vi "02.4 Transfering Data Through Queues.vi"() -> ()   [LabVIEW 2019]
uses:
  <extravilib>/ChannelInstances/Tag-bool.lvlib
panel:
  in  "Stop":bool
  in  "Process Speed Rate (%)":u32(slide) scale=10.0..200.0
  out "# of elements in Queue":i32
  out "Dequeued data":dbl
  in  "Enqueue Data":bool
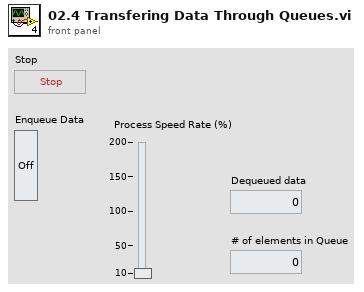
[diagram p1: front panel]
types:
  T1 = typedef "Tag-bool.lvlib/))Channel.ctl" = refnum<queue>
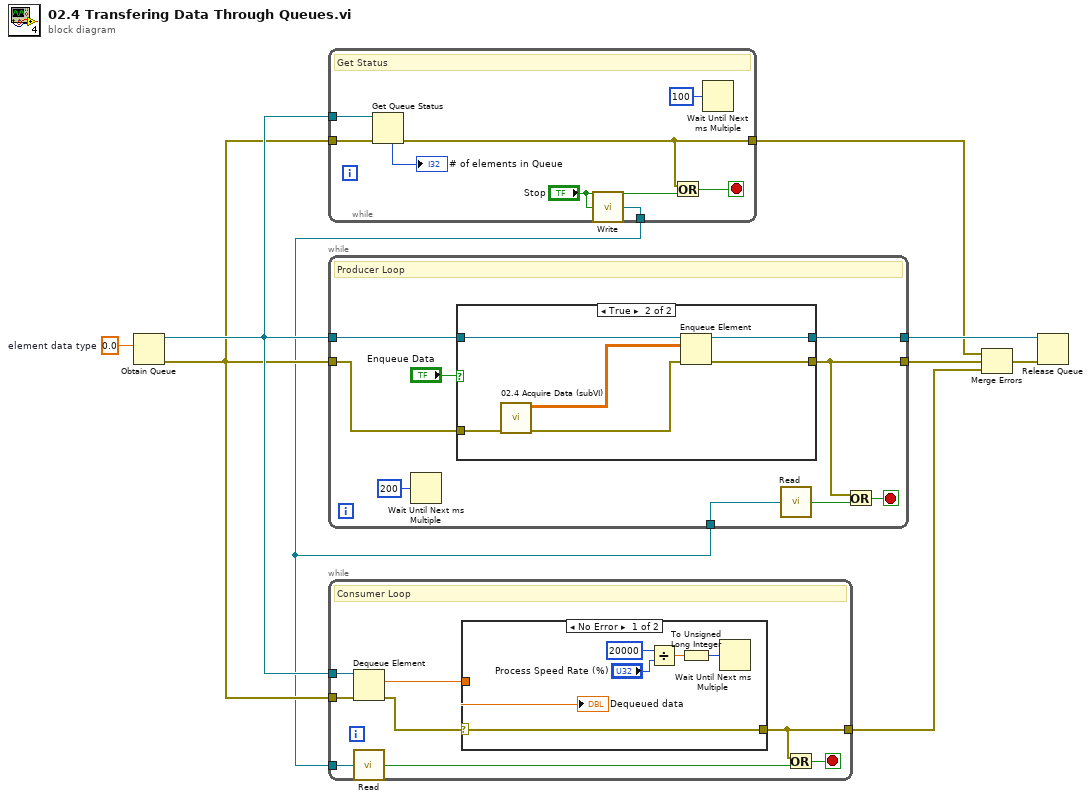
[diagram p0: block diagram]
diagram:
  w8 = 0.0  # element data type
  n1 = Obtain Queue(element data type=w8) -> (queue out=w7:refnum<queue>, error out=w6:errorcluster)  [unwired: 4 in, 1 out]
  n2 = while {
    tunnel: w7 -> [w17]
    tunnel: w6 -> [w16]
    tunnel: [w12] -> w4
    tunnel: [w10] -> w1
    stop <- w13 stop-if-true
    # "Get Status"
    n3 = Get Queue Status(queue=w17, error in (no error)=w16) -> (error out=w12:errorcluster, # elements in queue=→"# of elements in Queue":i32)  [unwired: 1 in, 6 out]
    n4 = call <extravilib>:"Write.vi"("element"="Stop") -> ("channel"=w10:T1)  [unwired: 1 out]
    n5 = Or(x=w12, y="Stop") -> (x .or. y?=w13:bool)
    n6 = Wait Until Next ms Multiple(millisecond multiple=u32 100 ("milliseconds to wait")) -> ()  [unwired: 1 out]
  }
  n7 = while {
    tunnel: w6 -> [w25]
    tunnel: [w21] -> w3
    tunnel: w7 -> [w26]
    tunnel: [w24] -> w9
    tunnel: w1 -> [w19]
    stop <- w22 stop-if-true
    # "Producer Loop"
    n8 = Wait Until Next ms Multiple(millisecond multiple=u32 200 ("milliseconds to wait")) -> ()  [unwired: 1 out]
    n9 = case shown="True" "Enqueue Data" {
      tunnel: w26 -> [w27 w34]
      tunnel: w25 -> [w28 w33]
      tunnel: [w27 w31] -> w24
      tunnel: [w28 w30] -> w21
      frame False {
      }
      frame True {
        n10 = call "02.4 Acquire Data (subVI).vi"("Error In"=w33) -> ("error out"=w32:errorcluster, "2D DBL"=w29:dbl[][])  [unwired: 9 in]
        n11 = Enqueue Element(queue=w34, element=w29, error in (no error)=w32) -> (queue out=w31:refnum<queue>, error out=w30:errorcluster)  [unwired: 1 in, 1 out]
      }
    }
    n12 = call <extravilib>:"Read.vi"("channel"=w19) -> ("element"=w18:bool)  [unwired: 1 in, 1 out]
    n13 = Or(x=w21, y=w18) -> (x .or. y?=w22:bool)
  }
  n14 = while {
    tunnel: w7 -> [w42]
    tunnel: w6 -> [w39]
    tunnel: [w36] -> w2
    tunnel: w1 -> [w38]
    stop <- w37 stop-if-true
    # "Consumer Loop"
    n15 = Dequeue Element(queue=w42, error in (no error)=w39) -> (element=w40:dbl, error out=w41:errorcluster)  [unwired: 1 in, 2 out]
    n16 = call <extravilib>:"Read.vi"("channel"=w38) -> ("element"=w35:bool)  [unwired: 1 in, 1 out]
    n17 = case shown="No Error" w41 {
      selector: w41 -> [w48 w49]
      tunnel: w40 -> [w47 _]
      tunnel: [w48 w49] -> w36
      frame No Error {
        n18 = Divide(x=u32 20000 ("y"), y="Process Speed Rate (%)") -> (x/y=w43:dbl)
        n19 = To Unsigned Long Integer(number=w43) -> (unsigned 32bit integer=w44:u32)
        n20 = Wait Until Next ms Multiple(millisecond multiple=w44) -> ()  [unwired: 1 out]
        "Dequeued data" <- w47
      }
      frame Error {
      }
    }
    n21 = Or(x=w36, y=w35) -> (x .or. y?=w37:bool)
  }
  n22 = Merge Errors(w4, w3, w2) -> (w5:errorcluster)
  n23 = Release Queue(queue=w9, error in (no error)=w5) -> ()  [unwired: 1 in, 3 out]
